vi "DataProcessLoadNewData XYGraph.vi"(0 "Graph":refnum<vi>, 5 "Graph":dbl[](array[numeric]), 7 "Pressure":dbl[](array[numeric]), 11 "error in (no error)":errorcluster) -> (4 "Graph Out":refnum<vi>, 15 "error out":errorcluster)   [LabVIEW 2013, in "main.lvlib"]
uses:
  main.lvlib
  Controls/Enum Variables.ctl
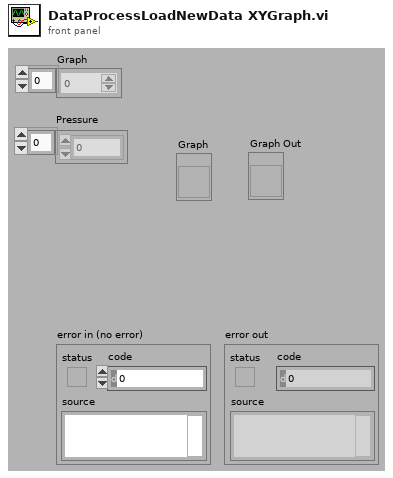
[diagram p1: front panel]
types:
  T1 = typedef "main.lvlib/Enum Variables.ctl" = enum16{"SetAcqFilter", "GetAcqFilter", "Set Filter", "Get Filter", "Set Height", "Get Height", "Set Blue Pressure", "Get Blue Pressure", "Set Red Pressure", "Get Red Pressure", "Init", "Reset Pressure", "Set Red Cursors", "Get Red Cursors", "Set Blue Cursors", "Get Blue Cursors", "Set Language", "Get Language", "Set Active Graphs", "Get ActiveGraphs", "Set Method", "Get Method", "Set Encryption", "Get Encryption", "Set ExcelVersion", "Get ExcelVersion", "Set DICOM Avail", "Get DICOM Avail", "Set DICOM Encode", "Get DICOM Encode", "Set JournalExport", "Get JournalExport", "Set Sequence", "Get Sequence", "Set DAQ Connected", "Get DAQ Connected", "Set Current Graph", "Get Current Graph", "Set General Settings", "Get Hyphenation", "Set Arm Calc Method", "Get Arm Calc Method", "Set Dicom Tags", "Get Dicom Tags", "Set BT Serial", "Get BT Serial", "Set BT Accepted Serials", "Get BT Accepted Serials", "Get BT License", "Set BT License"}
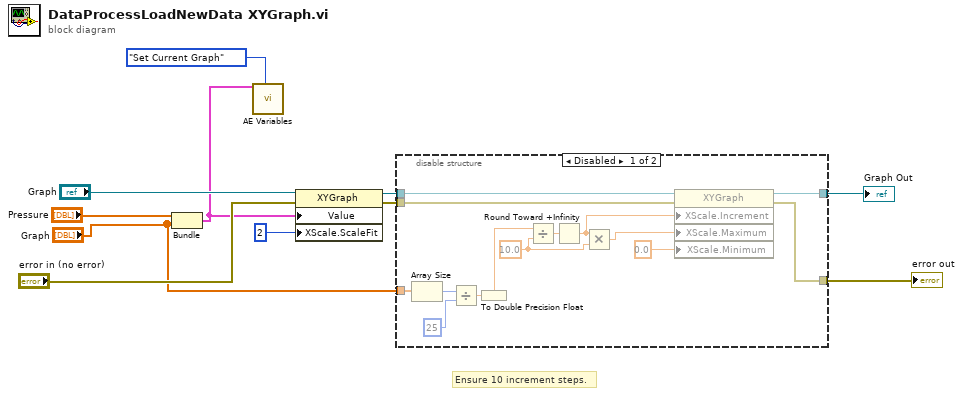
[diagram p0: block diagram]
diagram:
  # "Ensure 10 increment steps."
  n1 = Bundle("Pressure"="Pressure", "Graph"="Graph") -> (w1:cluster{"Pressure":dbl[], "Graph":dbl[]})  [unwired: 1 in]
  n2 = call "AE Variables.vi"("VariantIn"=w1, "Action"=Enum_Variables."Set Current Graph") -> ()  [unwired: 10 in, 8 out]
  n3 = property class="XYGraph"(reference="Graph", error in="error in (no error)", "Value"=w1, "XScale.ScaleFit"=u8 2 ("X Scale.Scale Fit")) -> (reference out=w6:refnum<vi>, error out=w5:errorcluster)
  n4 = disable-structure shown="Disabled" {
    disable-tunnel: [w21 w27] -> w10
    disable-tunnel: [w20 w26] -> w9
    disable-tunnel: w6 -> [w14 w27]
    disable-tunnel: w5 -> [w13 w26]
    disable-tunnel: "Graph" -> [w12 _]
    frame Disabled {
      w23 = 10.0 ("y")
      n5 = Array Size(array=w12) -> (size(s)=w19:i32)
      n6 = Divide(x=w19, y=25) -> (x/y=w17:dbl)
      n7 = To Double Precision Float(number=w17) -> (double precision float=w16:dbl)
      n8 = Divide(x=w16, y=w23) -> (x/y=w25:dbl)
      n9 = Round Toward +Infinity(x=w25) -> (ceil(x): smallest int >= x=w24:dbl)
      n10 = Multiply(x=w24, y=w23) -> (x*y=w22:dbl)
      n11 = property class="XYGraph"(reference=w14, error in=w13, "XScale.Increment"=w24, "XScale.Maximum"=w22, "XScale.Minimum"=0.0 ("X Scale.Range:Minimum")) -> (reference out=w21:refnum<vi>, error out=w20:errorcluster)
    }
    frame Enabled {
    }
  }
  "error out" <- w9
  "Graph Out" <- w10
